vi "VCS Set Master Encoder Parameter.vi"(0 "axis in":cluster{"keyHandle":u32, "nodeId":u16}={"keyHandle"=0, "nodeId"=1}, 5 "master encoder parameter":T1, 11 "error in (no error)":errorcluster) -> (4 "axis out":cluster{"keyHandle":u32, "nodeId":u16}={"keyHandle"=0, "nodeId"=1}, 15 "error out":errorcluster)   [LabVIEW 2010]
doc: "With function <B>VCS_SetMasterEncoderParameter</B> it is possible to write all parameters for master encoder mode."
uses:
  Resources/EposCmd.dll
  Resources/EposCmd64.dll
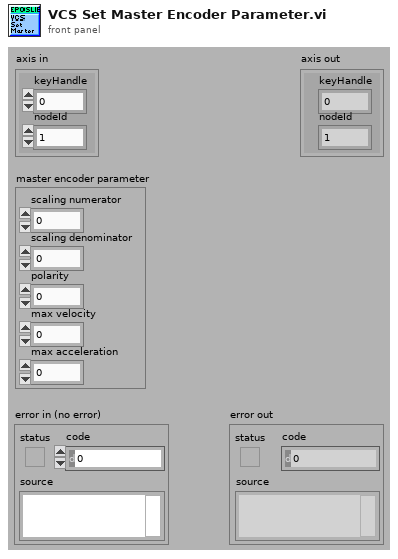
[diagram p1: front panel]
types:
  T1 = cluster{"scaling numerator":u16, "scaling denominator":u16, "polarity":u8, "max velocity":u32, "max acceleration":u32}
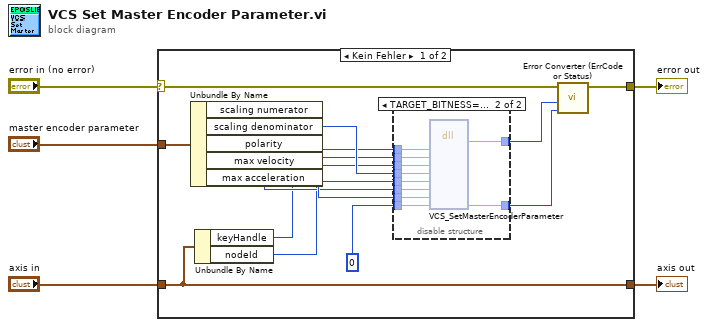
[diagram p0: block diagram]
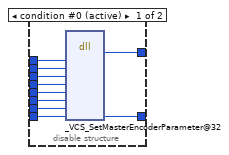
[diagram p2: hidden frame]
diagram:
  n1 = case shown="Kein Fehler" "error in (no error)" {
    selector: "error in (no error)" -> [w17 w40]
    tunnel: "axis in" -> [w19 w41]
    tunnel: [w19 w41] -> w4
    tunnel: [w18 w40] -> w3
    tunnel: "master encoder parameter" -> [w16 _]
    frame No Error {
      n2 = Unbundle By Name(w16) -> ("scaling numerator"=w11:u16, "scaling denominator"=w12:u16, "polarity"=w13:u8, "max velocity"=w14:u32, "max acceleration"=w15:u32)
      n3 = Unbundle By Name(w19) -> ("keyHandle"=w9:u32, "nodeId"=w10:u16)
      n4 = disable-structure shown="TARGET_BITNESS==64" {
        disable-tunnel: w15 -> [w29 w39]
        disable-tunnel: w14 -> [w28 w38]
        disable-tunnel: w13 -> [w27 w37]
        disable-tunnel: w12 -> [w26 w36]
        disable-tunnel: w11 -> [w25 w35]
        disable-tunnel: w10 -> [w24 w34]
        disable-tunnel: w9 -> [w23 w33]
        disable-tunnel: [w22 w32] -> w8
        disable-tunnel: [w21 w31] -> w7
        disable-tunnel: u32 0 ("pErrorCode") -> [w20 w30]
        frame condition #0 (active) {
          n5 = dll-call lib="C:/Sources/LabView/maxon EPOS/Resources/EposCmd.*" fn="_VCS_SetMasterEncoderParameter@32"("KeyHandle"=w23, "NodeId"=w24, "ScalingNumerator"=w25, "ScalingDenominator"=w26, "Polarity"=w27, "MaxVelocity"=w28, "MaxAcceleration"=w29, "pErrorCode"=w20) -> (w22:i32, "pErrorCode"=w21:u32)  [unwired: 10 in, 2 out]
        }
        frame condition #1 {
          n6 = dll-call lib="C:/setup/Resources/EposCmd64.*" fn="VCS_SetMasterEncoderParameter" ("EposCmd.dll:_VCS_SetMasterEncoderParameter@32")("KeyHandle"=w33, "NodeId"=w34, "ScalingNumerator"=w35, "ScalingDenominator"=w36, "Polarity"=w37, "MaxVelocity"=w38, "MaxAcceleration"=w39, "pErrorCode"=w30) -> ("Rückgabetyp"=w32:i32, "pErrorCode"=w31:u32)  [unwired: 10 in, 2 out]
        }
      }
      n7 = call "Error Converter (ErrCode or Status).vi"("error code"=w7, "return type"=w8, "error in (no error)"=w17) -> ("error out"=w18:errorcluster)  [unwired: 7 in]
    }
    frame Error {
    }
  }
  "error out" <- w3
  "axis out" <- w4
